vi "Diplom.vi"() -> ()   [LabVIEW 2018]
uses:
  VIs/TypeDef/States.ctl
  VIs/TypeDef/Diploma.ctl
  VIs/TypeDef/Settings.ctl
  <vilib>/Utility/miscctls.llb/LVPointTypeDef.ctl
  <vilib>/Utility/sysdir.llb/System Directory Type.ctl
  <vilib>/Utility/xml.llb/Read From XML File(string).vi
  <vilib>/Utility/xml.llb/Write to XML File(string).vi
  <vilib>/GPower/String/Library/GPString.lvlib
  <vilib>/GPower/Files & Folders/Library/GPFilesFolders.lvlib
panel:
  out "Selected Printer":string
  out "Svømmet ialt":dbl
  in  "PrintedDiplomasList":i32(listbox)
  in  "Stop Button":bool
  in  "Search":string
  in  "MemberList":i32[](listbox)
  # "Meter"
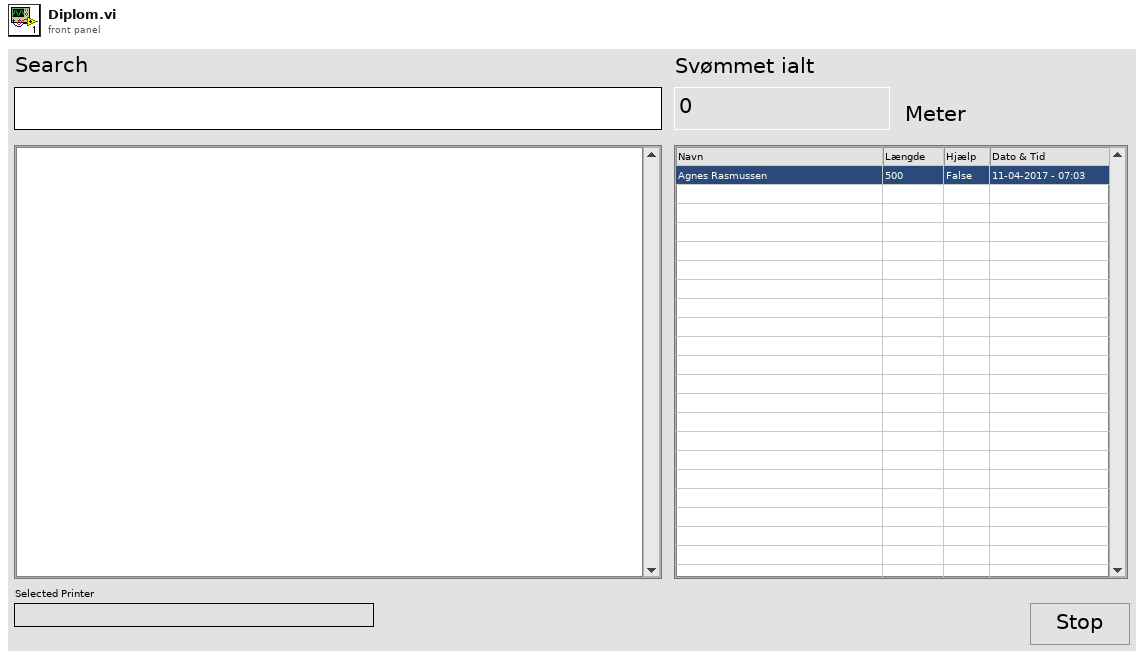
[diagram p1: front panel]
types:
  T1 = typedef "Settings.ctl" = cluster{"Printer":string}
  T2 = typedef "Diploma.ctl" = cluster{"Name":string, "Swim Length":string, "With Aids":bool, "Date":timestamp, "Unit":string}
  T3 = typedef "States.ctl" = enum16{"Init", "Event", "Preferences", "Update List", "Stop", "Error"}
  T4 = typedef "LVPointTypeDef.ctl" = cluster{"Horizontal":i16, "Vertical":i16}
  T5 = enum16{"open", "replace", "create", "open or create", "replace or create", "replace or create with confirmation"}
  T6 = typedef "System Directory Type.ctl" = i32
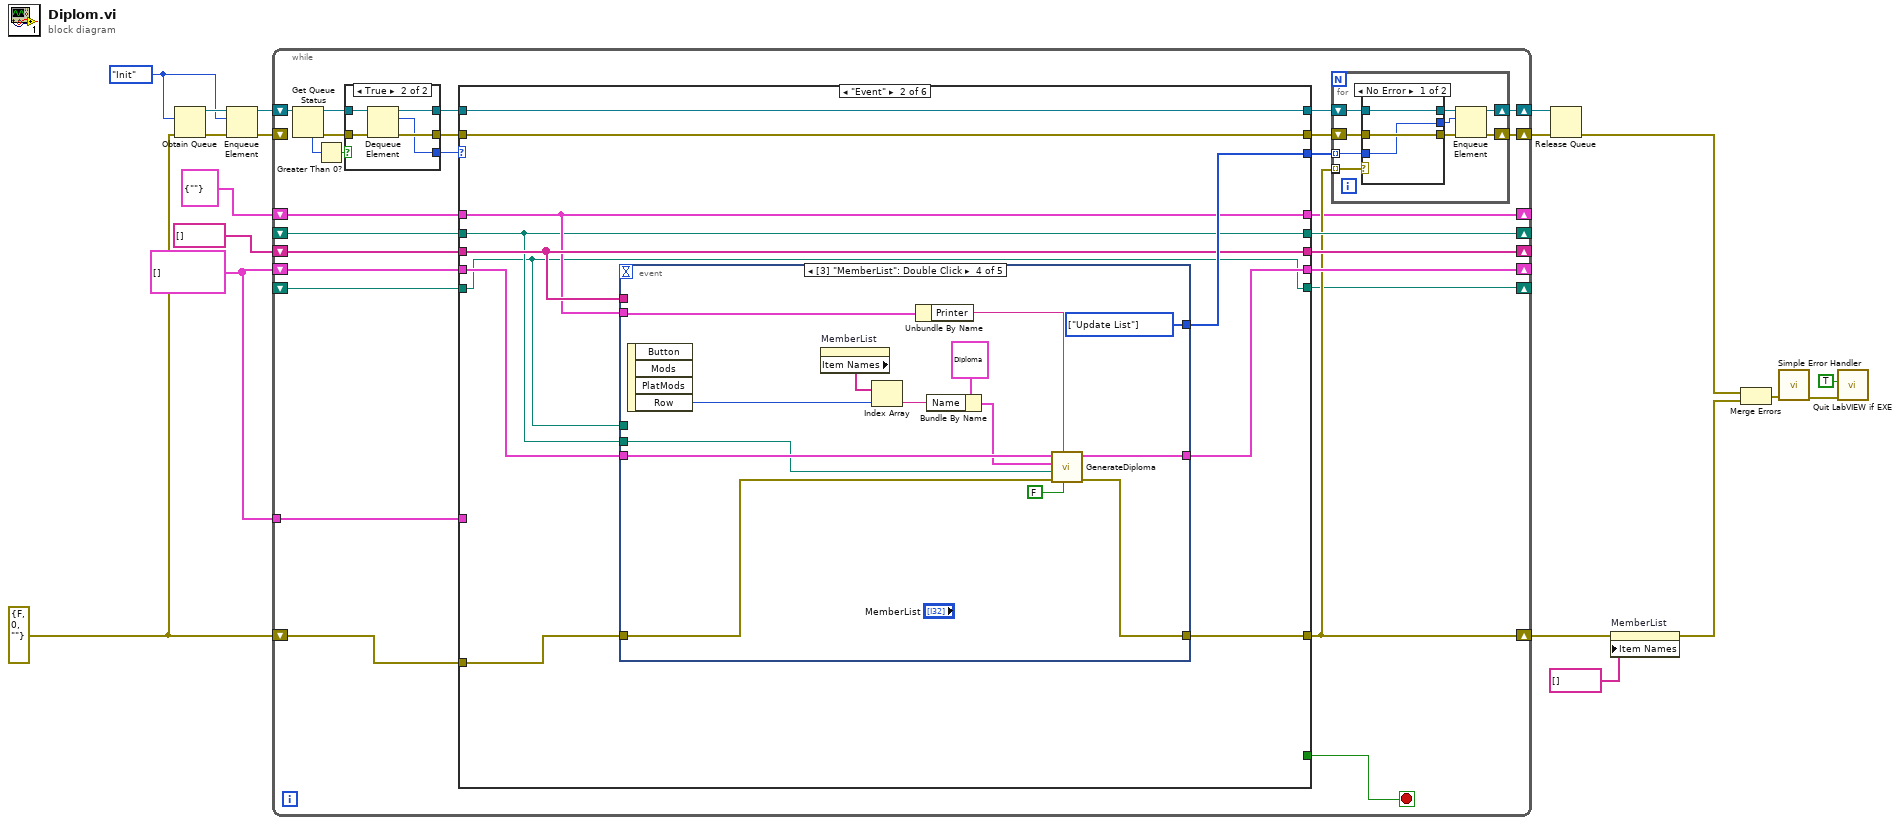
[diagram p0: block diagram]
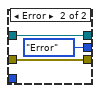
[diagram p2: hidden frame]
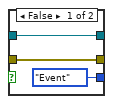
[diagram p3: hidden frame]
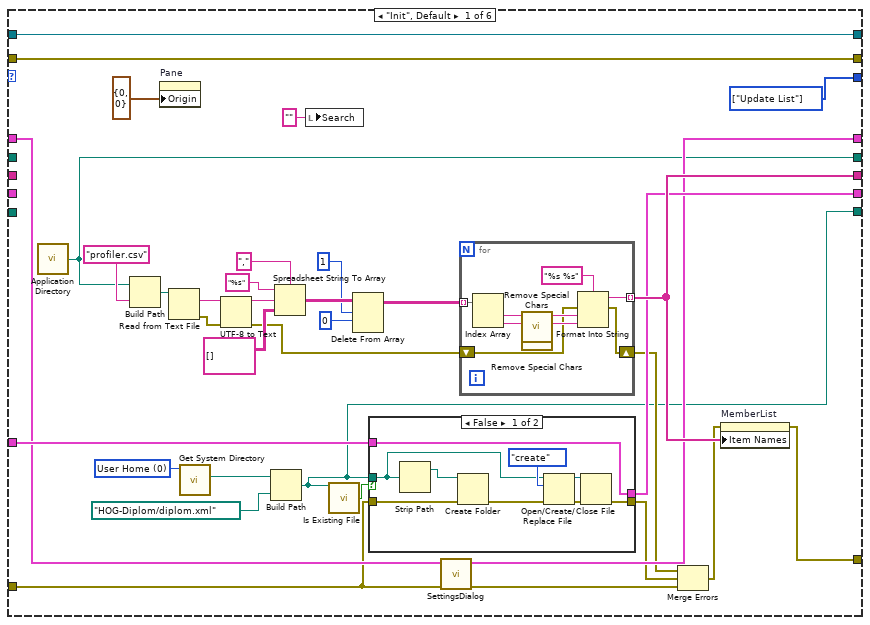
[diagram p4: hidden frame]
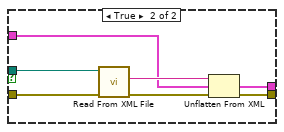
[diagram p5: hidden frame]
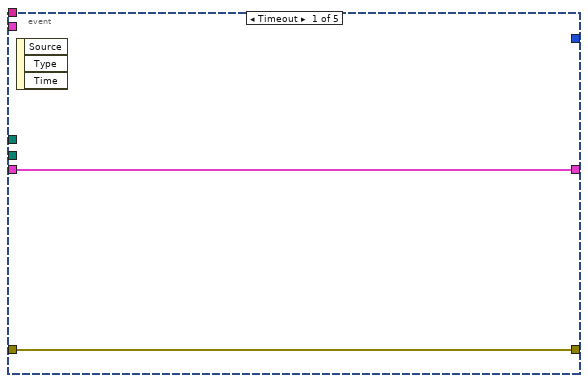
[diagram p6: hidden frame]
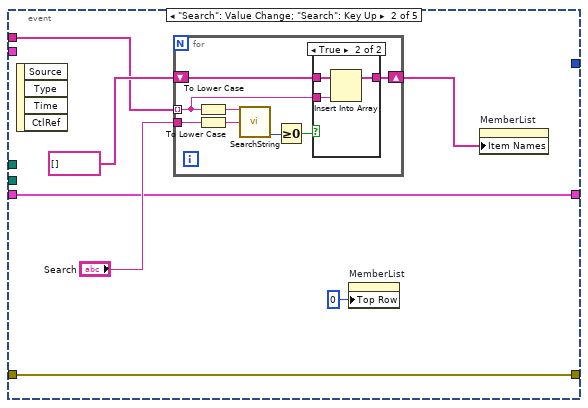
[diagram p7: hidden frame]
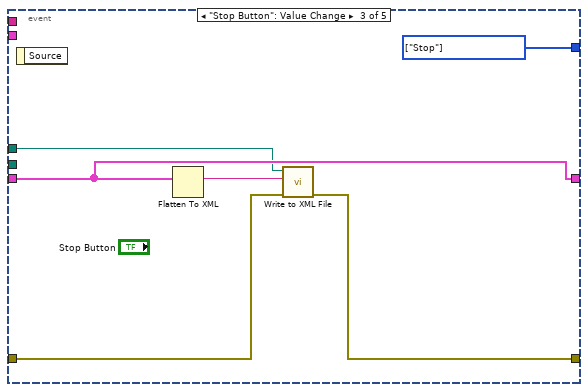
[diagram p9: hidden frame]
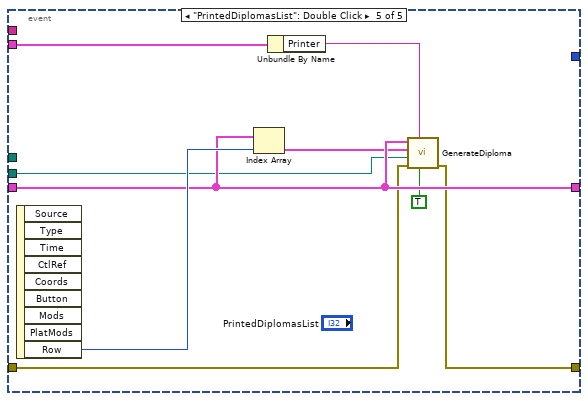
[diagram p10: hidden frame]
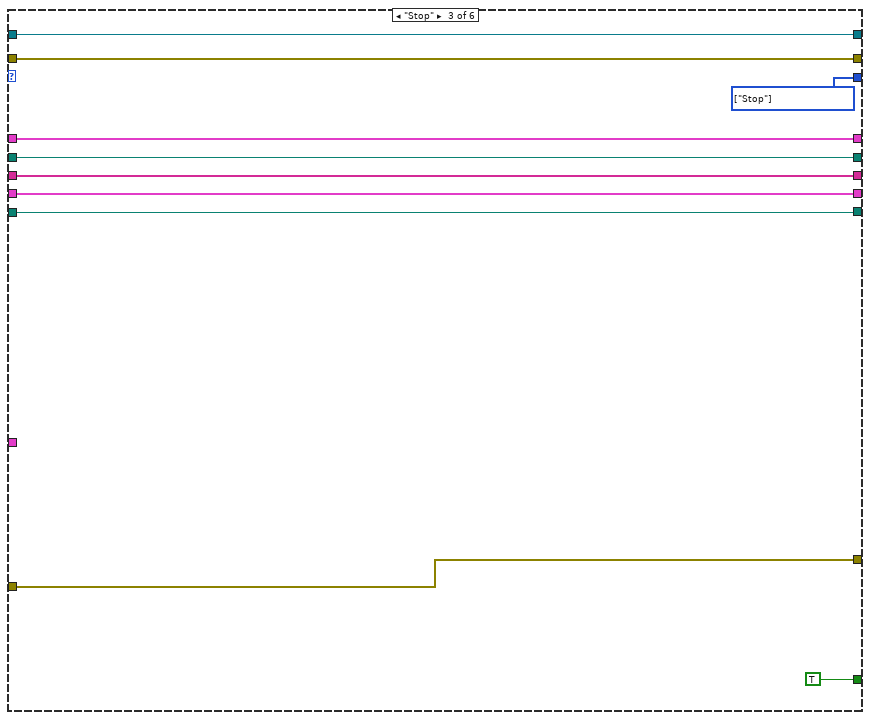
[diagram p11: hidden frame]
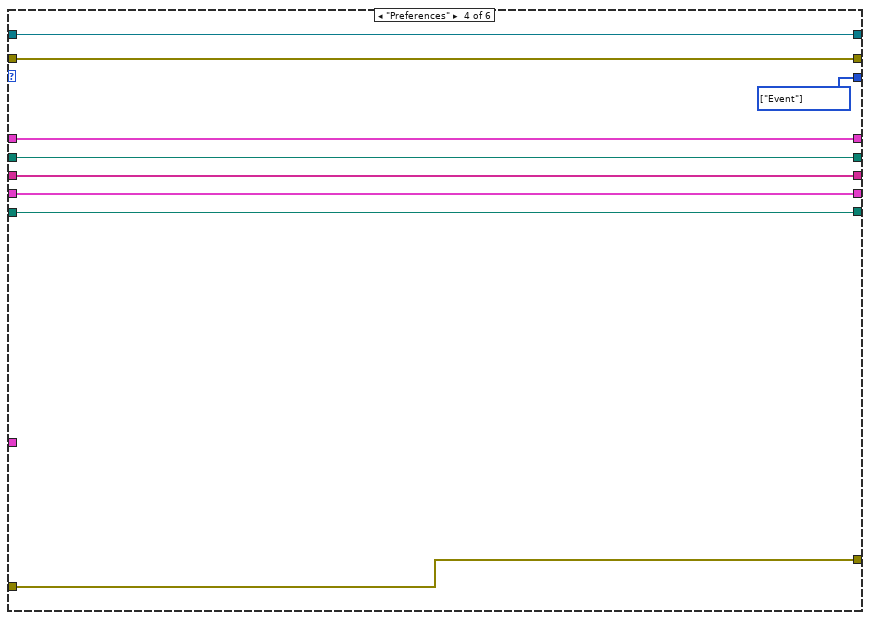
[diagram p12: hidden frame]
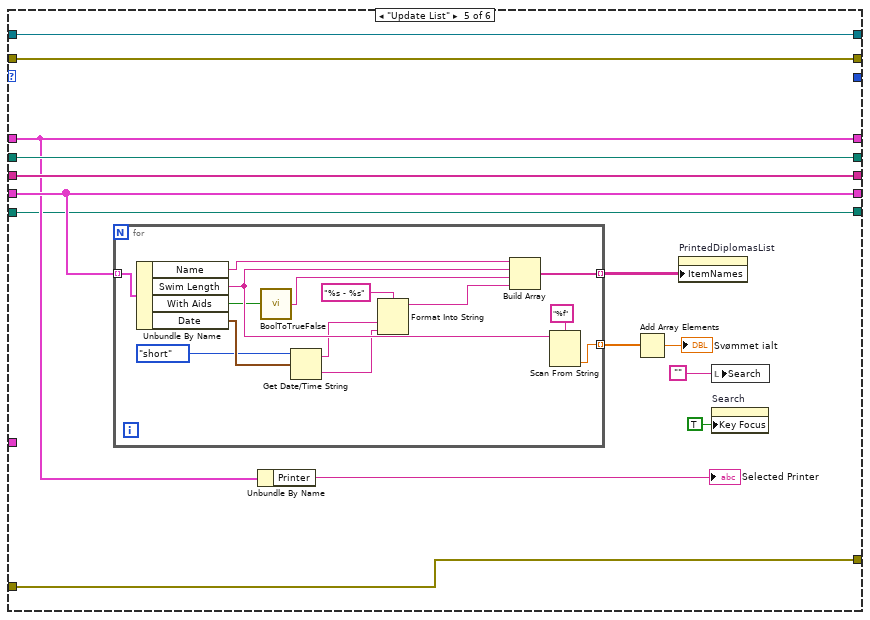
[diagram p13: hidden frame]
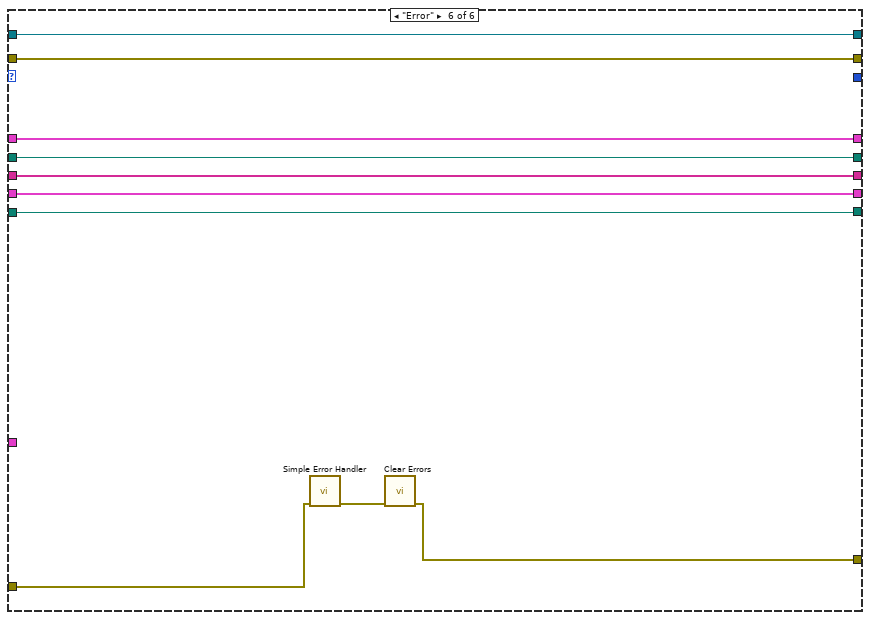
[diagram p14: hidden frame]
diagram:
  w1 = errorcluster {"status"=FALSE, "code"=0, "source"=""} ("error in (no error)")
  w10 = T2[] []
  w15 = States."Init"
  n1 = Obtain Queue(element data type=w15, error in (no error)=w1) -> (queue out=w18:refnum<queue>, error out=w17:errorcluster)  [unwired: 3 in, 1 out]
  n2 = Enqueue Element(queue=w18, element=w15, error in (no error)=w17) -> (queue out=w16:refnum<queue>, error out=w14:errorcluster)  [unwired: 1 in, 1 out]
  n3 = while {
    shift-right: [w32] -> w12
    shift-left: w14 -> [_]
    shift-right: [w33] -> w13
    shift-left: w16 -> [w41]
    shift-right: [w31] -> _
    shift-left: string[] [] -> [w30]
    shift-right: [w28] -> _
    shift-left: w10 -> [w29]
    shift-right: [w27] -> _
    shift-left: _ -> [w26]
    shift-right: [w24] -> w4
    shift-left: w1 -> [w25]
    tunnel: w10 -> [w23]
    shift-right: [w21] -> _
    shift-left: T1 {"Printer"=""} -> [w22]
    shift-right: [w20] -> _
    shift-left: _ -> [w19]
    stop <- w37 stop-if-true
    n4 = Get Queue Status(queue=w41) -> (queue out=w42:refnum<queue>, error out=w43:errorcluster, # elements in queue=w44:i32)  [unwired: 2 in, 5 out]
    n5 = Greater Than 0?(x=w44) -> (x > 0?=w45:bool)
    n6 = case shown="True" w45 {
      tunnel: w42 -> [w63 w67]
      tunnel: w43 -> [w62 w68]
      tunnel: [w63 w66] -> w40
      tunnel: [w62 w65] -> w39
      tunnel: [States."Event" w64] -> w38
      frame False {
      }
      frame True {
        n7 = Dequeue Element(queue=w67, error in (no error)=w68) -> (queue out=w66:refnum<queue>, element=w64:T3, error out=w65:errorcluster)  [unwired: 1 in, 1 out]
      }
    }
    n8 = case shown="\"Event\"" w38 {
      tunnel: w40 -> [w102 w139 w198 w207 w221 w245]
      tunnel: w39 -> [w103 w138 w199 w208 w222 w246]
      tunnel: [w103 w138 w199 w208 w222 w246] -> w36
      tunnel: [w102 w139 w198 w207 w221 w245] -> w35
      tunnel: [_ _ TRUE _ _ _] -> w37
      tunnel: [w101 w137 w196 w205 _ _] -> w34
      tunnel: [w100 w136 w195 w206 w220 w244] -> w31
      tunnel: w30 -> [_ w136 w195 w206 w220 w244]
      tunnel: w29 -> [_ w133 w194 w204 w217 w243]
      tunnel: [w95 w132 w194 w204 w217 w243] -> w28
      tunnel: [w75 w130 w193 w203 w219 w242] -> w27
      tunnel: w26 -> [_ w130 w193 w203 w219 w242]
      tunnel: w25 -> [w70 w135 w192 w202 w218 w240]
      tunnel: [w94 w134 w192 w202 w218 w239] -> w24
      tunnel: w23 -> [w96 _ _ _ _ _]
      tunnel: w22 -> [w92 w131 w191 w201 w211 w238]
      tunnel: [w93 w131 w191 w201 w211 w238] -> w21
      tunnel: [w69 w129 w190 w200 w209 w237] -> w20
      tunnel: w19 -> [_ w129 w190 w200 w209 w237]
      frame "Init", Default {
        w74 = T6 0 items=["User Home"=0, "User Desktop"=1, "User Documents"=2, "User Application Data"=3, "User Preferences"=4, "User Temporary"=5, "Public Documents"=6, "Public Application Data"=7, "Public Preferences"=8, "Public Cache"=13, "System Core Libraries"=9, "System Installed Libraries"=10, "Application Files"=11, "Boot Volume Root"=12] ("system directory type")
        w101 = T3[] [enum."Update List"] items=["Init", "Event", "Preferences", "Update List", "Stop", "Error"]
        n9 = call <vilib>:"Application Directory.vi"() -> ("Application Directory"=w75:path)
        n10 = Build Path(base path=w75, name or relative path="profiler.csv") -> (appended path=w82:path)
        n11 = property on="Pane" class="Pane"("Origin"=T4 {"Horizontal"=0, "Vertical"=0}) -> ()  [unwired: 2 in, 2 out]
        n12 = Read from Text File(file (use dialog)=w82) -> (text=w88:string, error out=w87:errorcluster)  [unwired: 3 in, 2 out]
        n13 = call <vilib>:"Get System Directory.vi"("system directory type"=w74) -> ("system directory"=w73:path)  [unwired: 10 in]
        n14 = UTF-8 to Text(8:w87, 11:w88) -> (0:w81:errorcluster, 3:w85:string)  [unwired: 1 in]
        n15 = Build Path(base path=w73, name or relative path=path "HOG-Diplom/diplom.xml") -> (appended path=w69:path)
        n16 = Spreadsheet String To Array(delimiter (Tab)=",", format string="%s", spreadsheet string=w85, array type (2D Dbl)=string[][] []) -> (array=w79:string[][])
        n17 = local write "Search"("" ("Search")) -> ()
        n18 = call <vilib>:"Is Existing File.vi"("File Path"=w69) -> ("Existing File?"=w71:bool)  [unwired: 4 in]
        n19 = Delete From Array(array=w79, length=1, index (row)=0) -> (array with subset deleted=w78:string[][])  [unwired: 1 in, 1 out]
        n20 = case shown="False" w71 {
          tunnel: w96 -> [w112 w118]
          tunnel: [w112 w116] -> w95
          tunnel: [w109 w115] -> w91
          tunnel: w70 -> [w107 w114]
          tunnel: w69 -> [w104 w113]
          frame False {
            n21 = Strip Path(path=w104) -> (stripped path=w105:path)  [unwired: 1 out]
            n22 = Create Folder(path (use dialog)=w105, error in=w107) -> (error out=w106:errorcluster)  [unwired: 1 in, 2 out]
            n23 = Open/Create/Replace File(file path (use dialog)=w104, error in=w106, operation (0:open)=T5."create") -> (refnum out=w108:refnum<file>, error out=w111:errorcluster)  [unwired: 3 in, 1 out]
            n24 = Close File(refnum=w108, error in=w111) -> (error out=w109:errorcluster)  [unwired: 1 out]
          }
          frame True {
            n25 = call-poly <vilib>:"Read From XML File.vi"("error in (no error)"=w114, "XML File Path"=w113) -> ("error out"=w117:errorcluster, "XML Elements"=w119:string)  [unwired: 7 in, 1 out]
            n26 = Unflatten From XML(xml string=w119, type=w118, error in (no error)=w117) -> (value=w116:T2[], error out=w115:errorcluster)
          }
        }
        n27 = call "SettingsDialog.vi"("error in (no error)"=w70, "Settings In"=w92) -> ("error out"=w90:errorcluster, "Settings Out"=w93:T1)  [unwired: 8 in]
        n28 = for {
          tunnel: [w123] -> w100 mode=indexing
          shift-right: [w121] -> w80
          shift-left: w81 -> [w122]
          tunnel: w78 -> [w120] mode=indexing
          n29 = Index Array(array=w120) -> (element #1=w128:string, element #2=w127:string)  [unwired: 2 in]
          n30 = call "Remove Special Chars.vi"("String in"=w128) -> ("String out"=w126:string)  [unwired: 8 in]
          n31 = call "Remove Special Chars.vi"("String in"=w127) -> ("String out"=w125:string)  [unwired: 8 in]
          n32 = Format Into String(format string="%s %s", error in=w122, w126, w125) -> (resulting string=w123:string, error out=w121:errorcluster)  [unwired: 1 in]
        }
        n33 = Merge Errors(w80, w91, w90) -> (w89:errorcluster)
        n34 = property on="MemberList" class="LstBox (strict)"(error in=w89, "Item Names"=w100) -> (error out=w94:errorcluster)  [unwired: 1 in, 1 out]
      }
      frame "Event" {
        n35 = event shown="[3] \"MemberList\": Double Click" {
          selector: _ -> [_ _ _ _ _]
          dyn-events: _ -> [_ _ _ _ _]
          timeout: _ -> [_ _ _ _ _]
          tunnel: [_ _ w166 w173 _] -> w137
          tunnel: w136 -> [_ w145 _ _ _]
          tunnel: w133 -> [w141 w144 w165 w178 w188]
          tunnel: w130 -> [_ _ _ w177 w187]
          tunnel: w135 -> [w140 w143 w163 w176 w186]
          tunnel: [w140 w143 w162 w175 w185] -> w134
          tunnel: [w141 w144 w165 w174 w188] -> w132
          tunnel: w131 -> [_ _ _ w169 w183]
          tunnel: w129 -> [_ _ w161 _ _]
          event Timeout {
            n36 = event-data() -> ()  [unwired: 1 in, 3 out]
          }
          event "Search": Value Change; "Search": Key Up {
            n37 = event-data() -> ()  [unwired: 1 in, 4 out]
            n38 = for {
              tunnel: "Search" -> [w151]
              shift-right: [w153] -> w146
              shift-left: string[] [] -> [w154]
              tunnel: w145 -> [w152] mode=indexing
              n39 = To Lower Case(string=w152) -> (all lower case string=w149:string)
              n40 = To Lower Case(string=w151) -> (all lower case string=w150:string)
              n41 = call <vilib>:"SearchString.vi"("String"=w149, "Search string"=w150) -> ("Offset past match"=w156:i32)  [unwired: 11 in, 2 out]
              n42 = Greater Or Equal To 0?(x=w156) -> (x >= 0?=w155:bool)
              n43 = case shown="True" w155 {
                tunnel: w154 -> [w157 w160]
                tunnel: [w157 w159] -> w153
                tunnel: w152 -> [_ w158]
                frame False {
                }
                frame True {
                  n44 = Insert Into Array(array=w160, new element=w158) -> (w159:string[])  [unwired: 1 in]
                }
              }
            }
            n45 = property on="MemberList" class="LstBox (strict)"("Top Row"=0) -> ()  [unwired: 2 in, 2 out]
            n46 = property on="MemberList" class="LstBox (strict)"("Item Names"=w146) -> ()  [unwired: 2 in, 2 out]
          }
          event "Stop Button": Value Change {
            w166 = T3[] [enum."Stop"] items=["Init", "Event", "Preferences", "Update List", "Stop", "Error"]
            n47 = event-data() -> ()  [unwired: 1 in, 1 out]
            n48 = Flatten To XML(anything=w165) -> (xml string=w164:string)
            n49 = call-poly <vilib>:"Write to XML File.vi"("error in (no error)"=w163, "XML Input"=w164, "XML File Path"=w161) -> ("error out"=w162:errorcluster)  [unwired: 6 in, 2 out]
          }
          event "MemberList": Double Click {
            w173 = T3[] [enum."Update List"] items=["Init", "Event", "Preferences", "Update List", "Stop", "Error"]
            n50 = event-data() -> ("Row"=w180:i32)  [unwired: 1 in, 3 out]
            n51 = property on="MemberList" class="LstBox (strict)"() -> ("Item Names"=w179:string[])  [unwired: 2 in, 2 out]
            n52 = Index Array(array=w179, index=w180) -> (element=w171:string)
            n53 = Unbundle By Name(w169) -> ("Printer"=w168:string)
            n54 = Bundle By Name(cluster=T2 {"Name"="", "Swim Length"="", "With Aids"=TRUE, "Date"=timestamp(0 s since 1904-01-01), "Unit"=""}, "Name"=w171) -> (w170:T2)
            n55 = call "GenerateDiploma.vi"("Reprint"=FALSE, "printer name (default)"=w168, "error in (no error)"=w176, "Path"=w177, "Diplom"=w170, "Diploma In"=w178) -> ("error out"=w175:errorcluster, "Diploma Out"=w174:T2[])  [unwired: 4 in]
          }
          event "PrintedDiplomasList": Double Click {
            n56 = event-data() -> ("Row"=w189:i32)  [unwired: 1 in, 8 out]
            n57 = Index Array(array=w188, index=w189) -> (element=w184:T2)
            n58 = Unbundle By Name(w183) -> ("Printer"=w182:string)
            n59 = call "GenerateDiploma.vi"("Reprint"=TRUE, "printer name (default)"=w182, "error in (no error)"=w186, "Path"=w187, "Diplom"=w184, "Diploma In"=w188) -> ("error out"=w185:errorcluster)  [unwired: 4 in, 1 out]
          }
        }
      }
      frame "Stop" {
        w196 = T3[] [enum."Stop"] items=["Init", "Event", "Preferences", "Update List", "Stop", "Error"]
      }
      frame "Preferences" {
        w205 = T3[] [enum."Event"] items=["Init", "Event", "Preferences", "Update List", "Stop", "Error"]
      }
      frame "Update List" {
        n60 = for {
          tunnel: w217 -> [w236] mode=indexing
          tunnel: [w234] -> w216 mode=indexing
          tunnel: [w231] -> w214 mode=indexing
          n61 = Unbundle By Name(w236) -> ("Name"=w235:string, "Swim Length"=w233:string, "With Aids"=w230:bool, "Date"=w228:timestamp)
          n62 = call <vilib>:"BoolToTrueFalse.vi"("Boolean"=w230) -> ("String"=w229:string)
          n63 = Get Date/Time String(date format (0)=enum16{"short", "long", "abbreviated"}."short", seconds (now)=w228) -> (date string=w226:string, time string=w225:string)  [unwired: 1 in]
          n64 = Format Into String(format string="%s - %s", w226, w225) -> (resulting string=w223:string)  [unwired: 2 in, 1 out]
          n65 = Build Array(w235, w233, w229, w223) -> (w234:string[])
          n66 = Scan From String(format string="%f", input string=w233) -> (output 1=w231:dbl)  [unwired: 3 in, 3 out]
        }
        n67 = Unbundle By Name(w211) -> ("Printer"=→"Selected Printer":string)
        n68 = Add Array Elements(numeric array=w214) -> (sum=→"Svømmet ialt":dbl)
        n69 = property on="PrintedDiplomasList" class="MCListbox (strict)"("ItemNames"=w216) -> ()  [unwired: 2 in, 2 out]
        n70 = local write "Search"("") -> ()
        n71 = property on="Search" class="Str"("Key Focus"=TRUE) -> ()  [unwired: 2 in, 2 out]
      }
      frame "Error" {
        n72 = call <vilib>:"Simple Error Handler.vi"("error in (no error)"=w240) -> ("error out"=w241:errorcluster)  [unwired: 4 in, 4 out]
        n73 = call <vilib>:"Clear Errors.vi"("error in (no error)"=w241) -> ("error out"=w239:errorcluster)  [unwired: 5 in, 1 out]
      }
    }
    n74 = for {
      shift-right: [w50] -> w32
      shift-left: w36 -> [w54]
      shift-right: [w49] -> w33
      shift-left: w35 -> [w53]
      tunnel: w34 -> [w52] mode=indexing
      tunnel: w24 -> [w51]
      tunnel: [w51] -> _ mode=indexing
      n75 = case shown="No Error" w51 {
        tunnel: w54 -> [w56 w59]
        tunnel: w53 -> [w57 w60]
        tunnel: w52 -> [w55 _]
        tunnel: [w57 w60] -> w48
        tunnel: [w56 w59] -> w47
        tunnel: [w55 States."Error"] -> w46
        frame No Error {
        }
        frame Error {
        }
      }
      n76 = Enqueue Element(queue=w48, element=w46, error in (no error)=w47) -> (queue out=w49:refnum<queue>, error out=w50:errorcluster)  [unwired: 1 in, 1 out]
    }
  }
  n77 = Release Queue(queue=w13, error in (no error)=w12) -> (error out=w9:errorcluster)  [unwired: 1 in, 2 out]
  n78 = property on="MemberList" class="LstBox (strict)"(error in=w4, "Item Names"=string[] []) -> (error out=w3:errorcluster)  [unwired: 1 in, 1 out]
  n79 = Merge Errors(w9, w3) -> (w8:errorcluster)
  n80 = call <vilib>:"Simple Error Handler.vi"("error in (no error)"=w8) -> ("error out"=w7:errorcluster)  [unwired: 4 in, 4 out]
  n81 = call "Quit LabVIEW if EXE.vi"("error in (no error)"=w7, "Quit LabVIEW?"=TRUE) -> ()  [unwired: 9 in, 1 out]
